vi "Get Validation Information.vi"(8 "error in (no error)":errorcluster, 11 "Routing and Faulting Custom Device Ref in":T3 format="%.0x") -> (0 "error out":errorcluster, 2 "Validation Information":T1, 3 "Routing and Faulting Custom Device Ref out":T3 format="%.0x")   [LabVIEW 2017, in "Routing and Faulting Scripting.lvlib"]
uses:
  Routing and Faulting Scripting.lvlib
  <vilib>/NI Veristand/Custom Device API/Custom Device Item Ref.ctl
  Validation Information.ctl
  Identifier Path Pair.ctl
  Shared/Routing and Faulting Hardware API/Routing and Faulting Hardware API.lvlib
  <vilib>/NI Veristand/Custom Device API/Custom Device API.lvlib
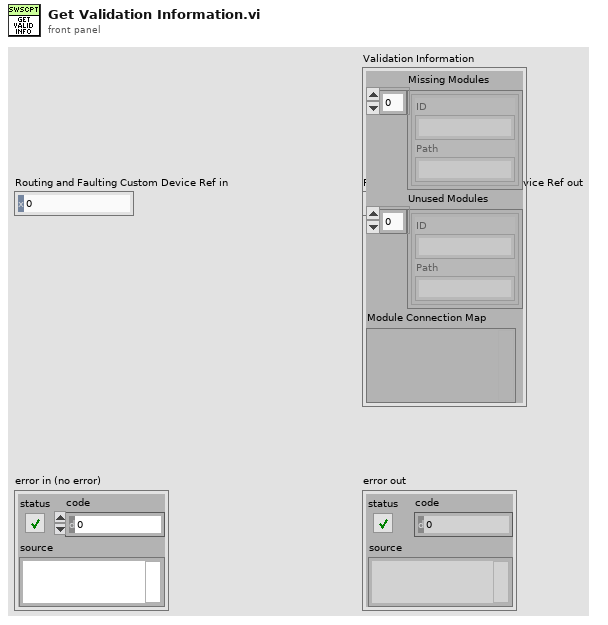
[diagram p1: front panel]
types:
  T1 = typedef "Routing and Faulting Scripting.lvlib/Validation Information.ctl" = cluster{"Missing Modules":T2[], "Unused Modules":T2[], "Module Connection Map":variant}
  T2 = typedef "Routing and Faulting Scripting.lvlib/Identifier Path Pair.ctl" = cluster{"ID":string, "Path":string}
  T3 = typedef "Custom Device API.lvlib/Custom Device Item Ref.ctl" = u64
  T4 = typedef "Routing and Faulting Hardware API.lvlib/Possible Connections for Endpoint.ctl" = cluster{"Source":string, "Destinations":string[]}
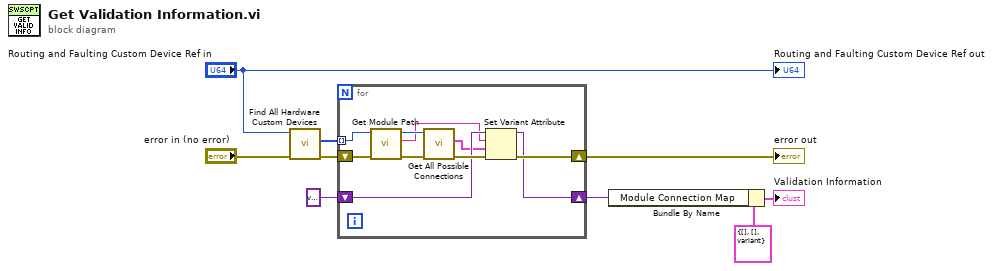
[diagram p0: block diagram]
diagram:
  n1 = call "Find All Hardware Custom Devices.vi"("error in (no error)"="error in (no error)", "Routing and Faulting Ref in"="Routing and Faulting Custom Device Ref in") -> ("error out"=w9:errorcluster, "Hardware Refs"=w8:T3[])  [unwired: 7 in, 1 out]
  n2 = for {
    shift-right: [w11] -> w4
    shift-left: w9 -> [w19]
    tunnel: w8 -> [w18] mode=indexing
    shift-right: [w10] -> w1
    shift-left: variant -> [w14]
    n3 = call "Get Module Path.vi"("error in (no error)"=w19, "Hardware Ref in"=w18) -> ("error out"=w16:errorcluster, "Module Path"=w12:string, "Hardware Ref out"=w17:T3)  [unwired: 6 in, 1 out]
    n4 = call "Get All Possible Connections.vi"("error in (no error)"=w16, "Hardware Ref in"=w17) -> ("error out"=w15:errorcluster, "Possible Connections"=w13:T4[])  [unwired: 6 in, 2 out]
    n5 = Set Variant Attribute(Variant=w14, name=w12, value=w13, error in=w15) -> (Variant out=w10:variant, error out=w11:errorcluster)  [unwired: 1 out]
  }
  "error out" <- w4
  n6 = Bundle By Name(cluster=T1 {"Missing Modules"=[], "Unused Modules"=[], "Module Connection Map"=variant} ("Validation Information"), "Module Connection Map"=w1) -> (→"Validation Information":T1)
  "Routing and Faulting Custom Device Ref out" <- "Routing and Faulting Custom Device Ref in"
